vi "extract_tone.vi"(7 "complex baseline":cdb, 8 "window":T1(ring)=enum."Hanning", 9 "tone frequency [Hz]":dbl=1000.0 format="%.2f", 10 "df":dbl, 11 "complex fft":cdb[](array[numeric])) -> (2 "phase (rad)":dbl format="%#_3p", 3 "amplitude":dbl format="%#_3p")   [LabVIEW 2021]
uses:
  <vilib>/Analysis/baseanly.llb/Complex Dot Product.vi
  <vilib>/Analysis/NI_AALBase.lvlib
panel:
  out "x < y?":bool
  out "size(s)":i32
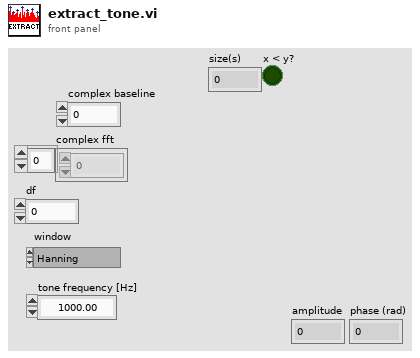
[diagram p1: front panel]
types:
  T1 = enum16{"None ", "Hanning", "Hamming", "Blackman-Harris", "Exact Blackman", "Blackman", "Flat Top", "4 Term B-Harris ", "7 Term B-Harris", "Low Sidelobe"}
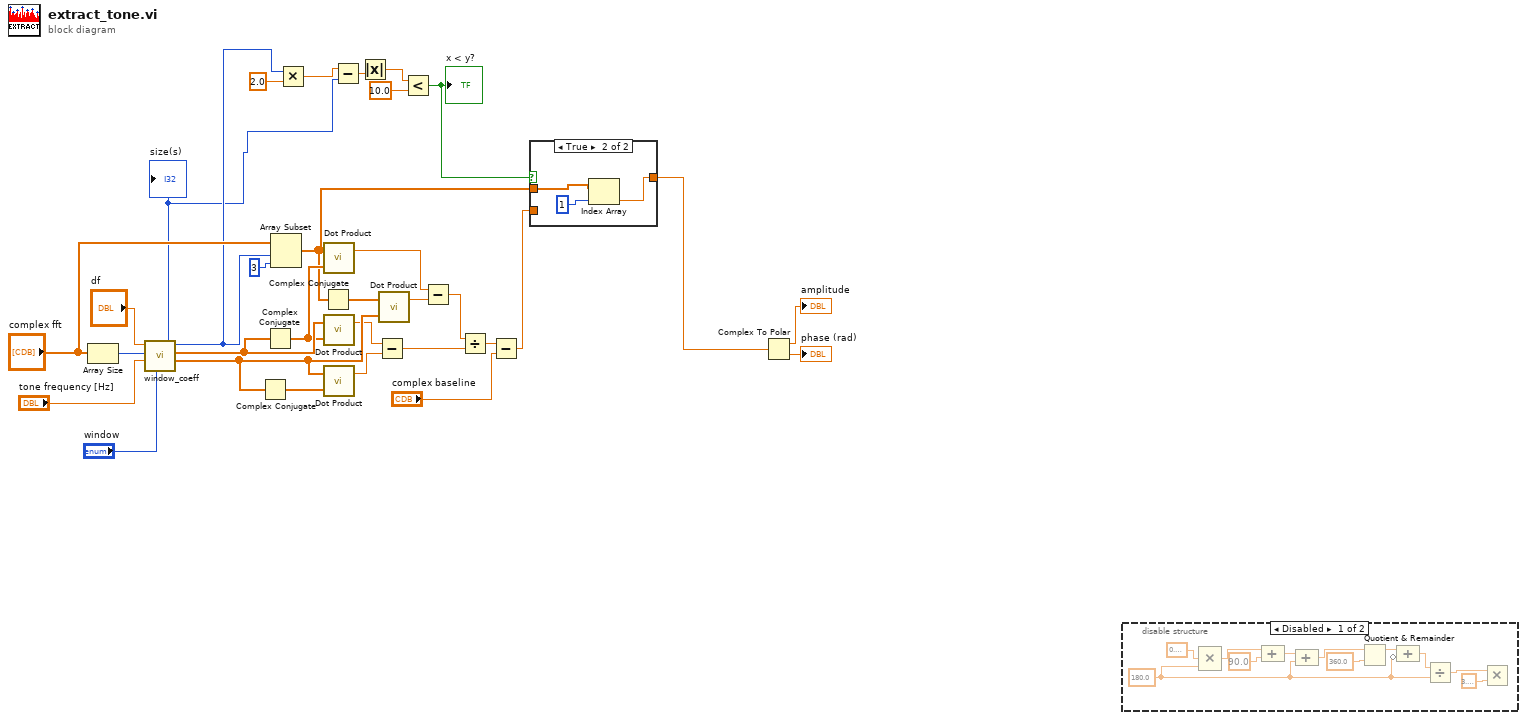
[diagram p0: block diagram]
diagram:
  n1 = Array Size(array="complex fft") -> (size(s)=w8:i32)
  "size(s)" <- w8
  n2 = call "window_coeff.vi"("window"="window", "tone frequency [Hz]"="tone frequency [Hz]", "Numeric in"=w8, "df"="df") -> ("Array 2"=w28:cdb[], "Array"=w23:cdb[], "Numeric out"=w10:i32)  [unwired: 5 in]
  n3 = Complex Conjugate(1:w28) -> (0:w20:cdb[])
  n4 = Complex Conjugate(1:w23) -> (0:w21:cdb[])
  n5 = Array Subset(array="complex fft", index=w10, length=3) -> (w3:cdb[])
  n6 = Multiply(x=w10, y=2.0) -> (x*y=w9:dbl)
  n7 = Complex Conjugate(1:w3) -> (0:w22:cdb[])
  n8 = call-poly <vilib>:"Dot Product.vi"("Y Vector"=w21, "X Vector"=w3) -> ("X * Y"=w24:cdb)  [unwired: 1 out]
  n9 = call-poly <vilib>:"Dot Product.vi"("Y Vector"=w21, "X Vector"=w23) -> ("X * Y"=w25:cdb)  [unwired: 1 out]
  n10 = call-poly <vilib>:"Dot Product.vi"("Y Vector"=w20, "X Vector"=w28) -> ("X * Y"=w19:cdb)  [unwired: 1 out]
  n11 = Subtract(x=w9, y=w8) -> (x-y=w6:dbl)
  n12 = Absolute Value(x=w6) -> (abs(x)=w5:dbl)
  n13 = Subtract(x=w25, y=w19) -> (x-y=w27:cdb)
  n14 = call-poly <vilib>:"Dot Product.vi"("Y Vector"=w28, "X Vector"=w22) -> ("X * Y"=w29:cdb)  [unwired: 1 out]
  n15 = Less?(x=w5, y=10.0) -> (x < y?=w4:bool)
  "x < y?" <- w4
  n16 = Subtract(x=w24, y=w29) -> (x-y=w26:cdb)
  n17 = Divide(x=w26, y=w27) -> (x/y=w13:cdb)
  n18 = Subtract(x=w13, y="complex baseline") -> (x-y=w2:cdb)
  n19 = case shown="True" w4 {
    tunnel: w3 -> [_ w34]
    tunnel: w2 -> [w32 _]
    tunnel: [w32 w33] -> w1
    frame False {
    }
    frame True {
      n20 = Index Array(array=w34, index=1) -> (element=w33:cdb)
    }
  }
  n21 = Complex To Polar(r * e^(i*theta)=w1) -> (r=→"amplitude":dbl, theta=→"phase (rad)":dbl)
  n22 = disable-structure shown="Disabled" {
    frame Disabled {
      w38 = 180.0 ("Input")
      n23 = Compound Arithmetic op=MULTIPLY(0.3183098861837907, w38) -> (w45:dbl)  [unwired: 1 in]
      n24 = Compound Arithmetic op=ADD(w45, 90.0 ("value")) -> (w44:dbl)
      n25 = Compound Arithmetic op=ADD(w44, w38) -> (w43:dbl)
      n26 = Quotient & Remainder(x=w43, y=360.0 ("value")) -> (x-y*floor(x/y)=w41:dbl)  [unwired: 1 out]
      n27 = Compound Arithmetic op=ADD(w41, invert w38) -> (w39:dbl)
      n28 = Divide(x=w39, y=w38) -> (x/y=w37:dbl)
      n29 = Multiply(x=w37, y=3.141592653589793) -> ()  [unwired: 1 out]
    }
    frame Enabled {
    }
  }
